vi "Fix Velocities from Joysticks.vi"(10 "Axes":dbl[](array[numeric]), 11 "Deadband":cluster{"value":dbl, "value":dbl, "value":dbl}) -> (1 "Sending Input?":bool, 2 "Adjusted Robot Velocities":T1)   [LabVIEW 2023]
uses:
  swerve/Type Definitions/Data/Robot Velocities.ctl
  <vilib>/Rock Robotics/WPI/Joystick/XBox Axes Indexer.ctl
  3ad3cf1c-8863-4f6c-a2e6-a00d4e593ecd.vi
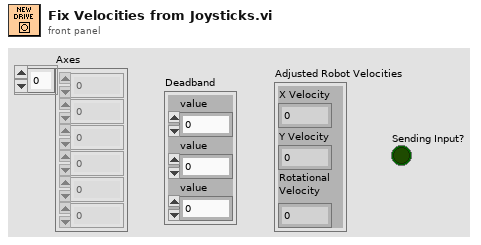
[diagram p1: front panel]
types:
  T1 = typedef "Robot Velocities.ctl" = cluster{"X Velocity":dbl, "Y Velocity":dbl, "Rotational \nVelocity":dbl}
  T2 = typedef "XBox Axes Indexer.ctl" = enum16{"Left X", "Left Y", "Left Trigger", "Right Trigger", "Right X", "Right Y"}
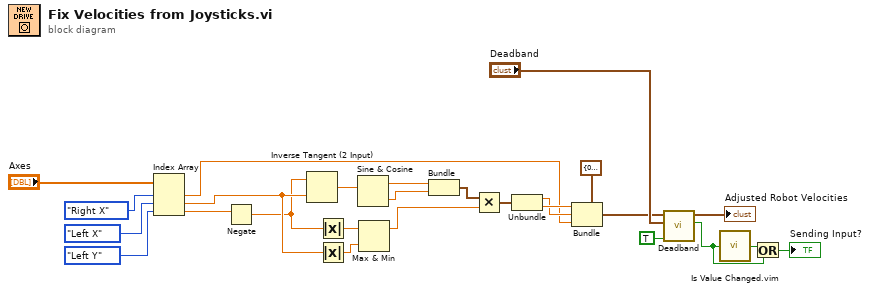
[diagram p0: block diagram]
diagram:
  n1 = Index Array(array="Axes", index #1=XBox_Axes_Indexer."Right X" ("XBox Axes"), index #2=XBox_Axes_Indexer."Left X" ("XBox Axes"), index #3=XBox_Axes_Indexer."Left Y" ("XBox Axes")) -> (element #1=w1:dbl, element #2=w18:dbl, element #3=w14:dbl)
  n2 = Negate(x=w14) -> (-x=w13:dbl)
  n3 = Inverse Tangent (2 Input)(1:w18, 2:w13) -> (0:w10:dbl)
  n4 = Absolute Value(x=w13) -> (abs(x)=w7:dbl)
  n5 = Absolute Value(x=w18) -> (abs(x)=w6:dbl)
  n6 = Sine & Cosine(0:w10) -> (1:w9:dbl, 2:w8:dbl)
  n7 = Max & Min(x=w7, y=w6) -> (max(x,y)=w4:dbl)  [unwired: 1 out]
  n8 = Bundle(w9, w8) -> (w5:cluster{dbl, dbl})  [unwired: 1 in]
  n9 = Multiply(x=w5, y=w4) -> (x*y=w3:cluster{dbl, dbl})
  n10 = Unbundle(w3) -> (w2:dbl, w11:dbl)
  n11 = Bundle(cluster=cluster{dbl, dbl, "upper limit":dbl} {0.0, 0.0, "upper limit"=0.0}, w11, w2, "upper limit"=w1) -> (w20:cluster{dbl, dbl, "upper limit":dbl})
  n12 = call "Deadband.vi"("Rescaling On?"=TRUE, "Deadband Info"="Deadband", "Robot Velocities"=w20) -> ("Sending Input?"=w16:bool, "Adjusted Robot Velocities"=→"Adjusted Robot Velocities":T1)  [unwired: 7 in]
  n13 = call "Is Value Changed.vim"("value"=w16) -> ("changed or first call?"=w17:bool)
  n14 = Or(x=w17, y=w16) -> (x .or. y?=→"Sending Input?":bool)
